vi "CrossDir.vi"(11 "View":i32[](array[numeric]) caption="View (Team Index, -1: empty)") -> (2 "ValidDir":bool, 3 "Direction":T1=enum."N")   [LabVIEW 2017, in "Atom.lvclass"]
uses:
  Atom.lvclass
  Type Defs/Direction Enum.ctl
  Type Defs/SB Type Defs.lvlib
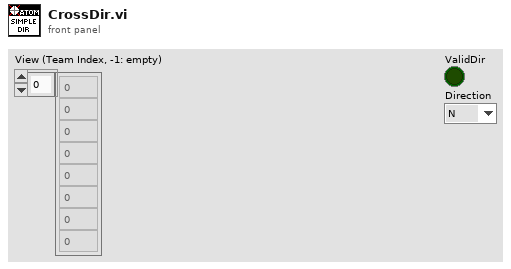
[diagram p1: front panel]
types:
  T1 = typedef "SB Type Defs.lvlib/Direction Enum.ctl" = enum16{"NW", "N", "NE", "E", "SE", "S", "SW", "W"}
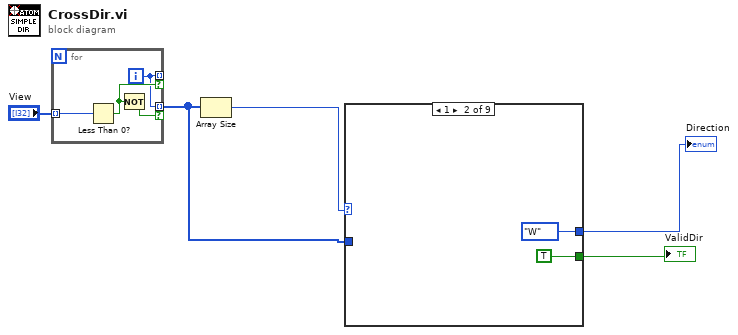
[diagram p0: block diagram]
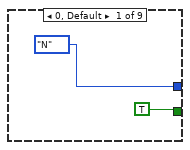
[diagram p2: hidden frame]
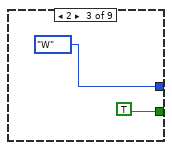
[diagram p3: hidden frame]
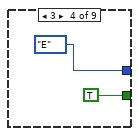
[diagram p4: hidden frame]
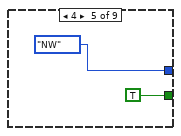
[diagram p5: hidden frame]
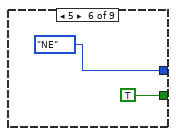
[diagram p6: hidden frame]
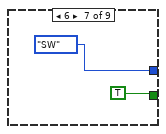
[diagram p7: hidden frame]
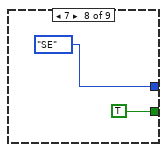
[diagram p8: hidden frame]
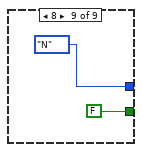
[diagram p9: hidden frame]
diagram:
  n1 = for {
    tunnel: "View" -> [w9] mode=indexing
    tunnel: [w7] -> _ mode=indexing if=w8
    tunnel: [w7] -> w2 mode=indexing if=w6
    i -> [w7]
    n2 = Less Than 0?(x=w9) -> (x < 0?=w8:bool)
    n3 = Not(x=w8) -> (.not. x?=w6:bool)
  }
  n4 = Array Size(array=w2) -> (size(s)=w4:i32)
  n5 = case shown="1" w4 {
    tunnel: [TRUE TRUE TRUE TRUE TRUE TRUE TRUE TRUE FALSE] -> w3
    tunnel: w2 -> [_ _ _ _ _ _ _ _ _]
    tunnel: [Direction_Enum."N" ("Direction") Direction_Enum."W" ("Direction") Direction_Enum."W" ("Direction") Direction_Enum."E" ("Direction") Direction_Enum."NW" ("Direction") Direction_Enum."NE" ("Direction") Direction_Enum."SW" ("Direction") Direction_Enum."SE" ("Direction") Direction_Enum."N" ("Direction")] -> w1
    frame 0, Default {
    }
    frame 1 {
    }
    frame 2 {
    }
    frame 3 {
    }
    frame 4 {
    }
    frame 5 {
    }
    frame 6 {
    }
    frame 7 {
    }
    frame 8 {
    }
  }
  "ValidDir" <- w3
  "Direction" <- w1
